vi "5. Identification.vi"() -> ()   [LabVIEW 2019, in "SJCube.lvlib"]
uses:
  SJCube.lvlib
  idState.ctl
  <vilib>/Platform/TimedLoop/XDataNode/timing_clust.ctl
  <vilib>/Platform/TimedLoop/XDataNode/nitl_modes.ctl
  <vilib>/Platform/TimedLoop/XDataNode/wakeup.ctl
  <vilib>/Platform/TimedLoop/XDataNode/XDataNode.xnode
  <vilib>/Platform/TimedLoop/XDataNode/XDNodeRunTimeDep.lvlib
panel:
  in  "Logging Setting":T1
  out "motor overswing":bool
  in  "overswing (deg)":dbl=15.0 format="%#_13g"
  out "Stick deg greater then":bool
  out "error out":errorcluster
  in  "Play Button":bool
  out "Waveform Chart":T2(graph)
  in  "Configuration Sine":T3={"Amp (Volts)"=0.4, "Freq (Hz)"=10.0, "Time (s)"=5.0, "SignalType"=enum."IdSine"} {"Amp (Volts)" scale=0.0..12.0}
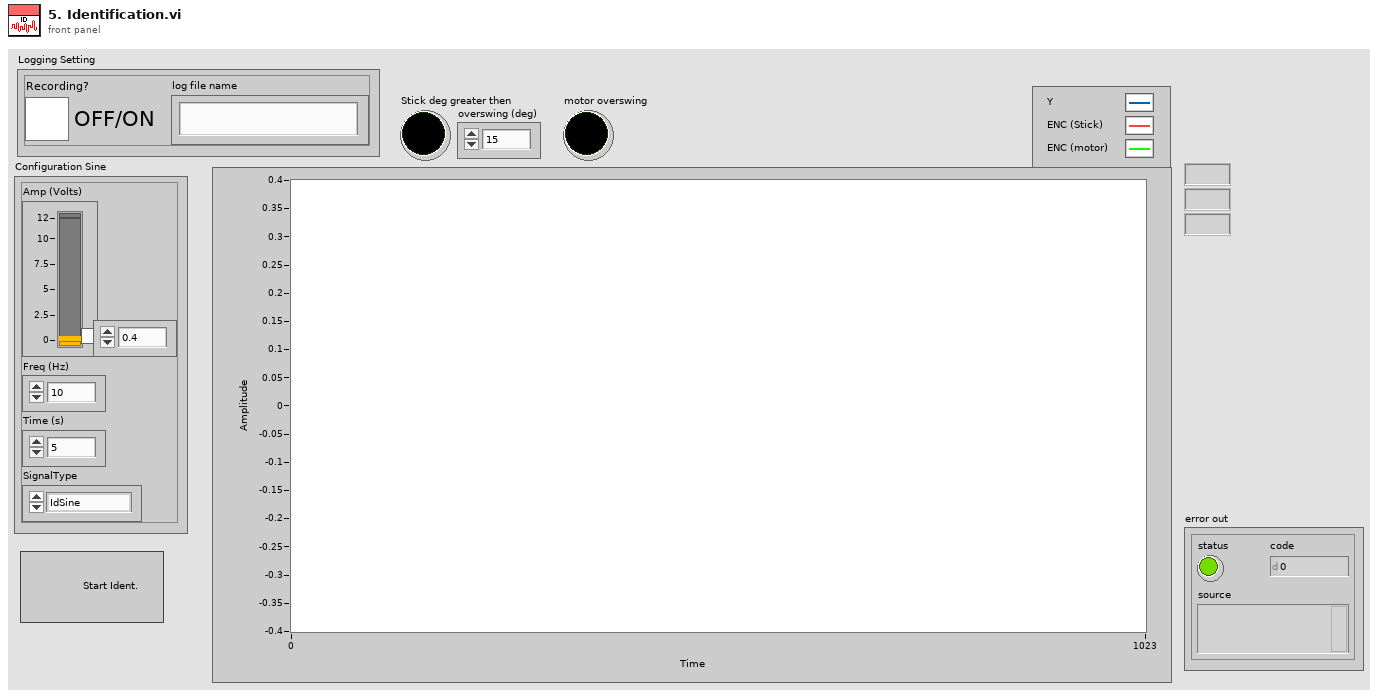
[diagram p1: front panel]
types:
  T1 = cluster{"Recording?":bool, "log file name":string}
  T2 = cluster{dbl, "StickEncoder (deg)":dbl, "MotorEncoder (deg)":dbl}
  T3 = cluster{"Amp (Volts)":dbl, "Freq (Hz)":dbl, "Time (s)":dbl, "SignalType":enum16{"IdSine", "IdSquare"}}
  T4 = typedef "SJCube.lvlib/idState.ctl" = enum16{"Configuration", "Id", "Logging", "End"}
  T5 = cluster{dbl, "StickEncoder (deg)":dbl, "MotorEncoder (deg)":dbl}[]
  T6 = typedef "XDNodeRunTimeDep.lvlib/timing_clust.ctl" = cluster{"Expected End [f-1]":u64, "Actual End [f-1]":u64, "Finished Late? [f-1]":bool, "Expected End [i-1]":u64, "Actual End [i-1]":u64, "Finished Late? [i-1]":bool, "Expected Start [i]":u64, "Actual Start [i]":u64, "Expected Start [f]":u64, "Actual Start [f]":u64, "Source Name":string, "Structure Name":string, "Period":i64, "Deadline":i64, "Offset":i64, "Start":i64, "Priority":i32, "Timeout":i32, "Mode":T7, "Wakeup Reason":T8, "Error":errorcluster, "Source Type":string, "Secondary Source Type":string, "Global End Time":u64, "Global Start Time":u64, "Frame Duration":u64, "Iteration Duration":u64, "Assigned CPU":i32, "I/O Scan Engine Mode":u32}
  T7 = typedef "XDNodeRunTimeDep.lvlib/nitl_modes.ctl" = enum32{"No Change", "Process missed periods, maintain original phase", "Discard missed periods, maintain original phase", "Process missed periods, ignore original phase", "Discard missed periods, ignore original phase"}
  T8 = typedef "XDNodeRunTimeDep.lvlib/wakeup.ctl" = enum32{"Normal", "Aborted", "Asynchronous wakeup", "Timing source error", "Timed loop error", "Timeout"}
  T9 = enum16{"open", "replace", "create", "open or create", "replace or create", "replace or create with confirmation"}
  T10 = cluster{"Amp (Volts)":dbl, "StickEncoder (deg)":dbl, "MotorEncoder (deg)":dbl}
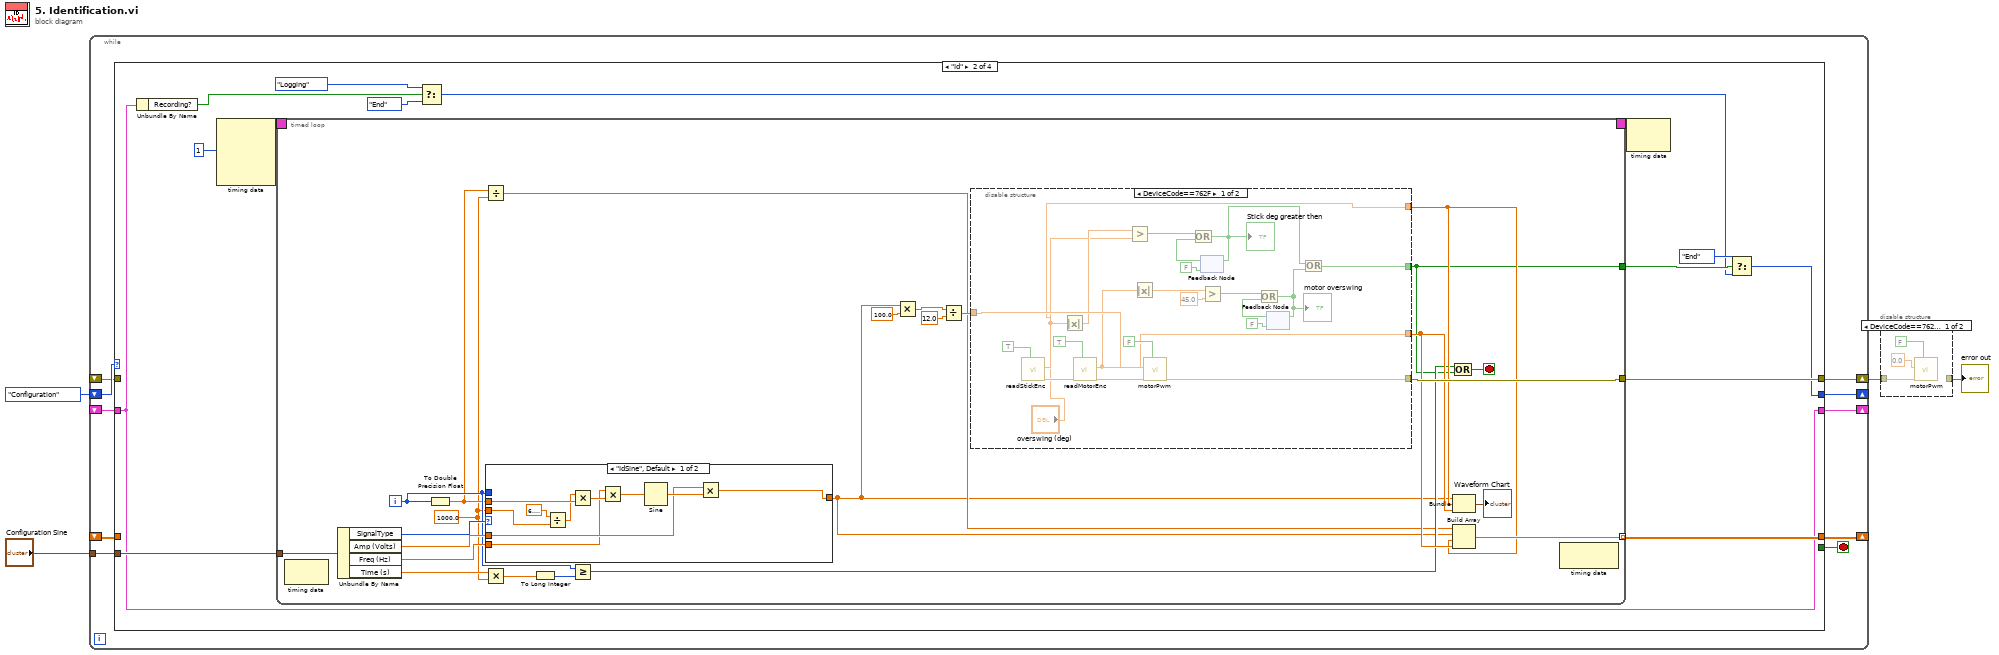
[diagram p0: block diagram]
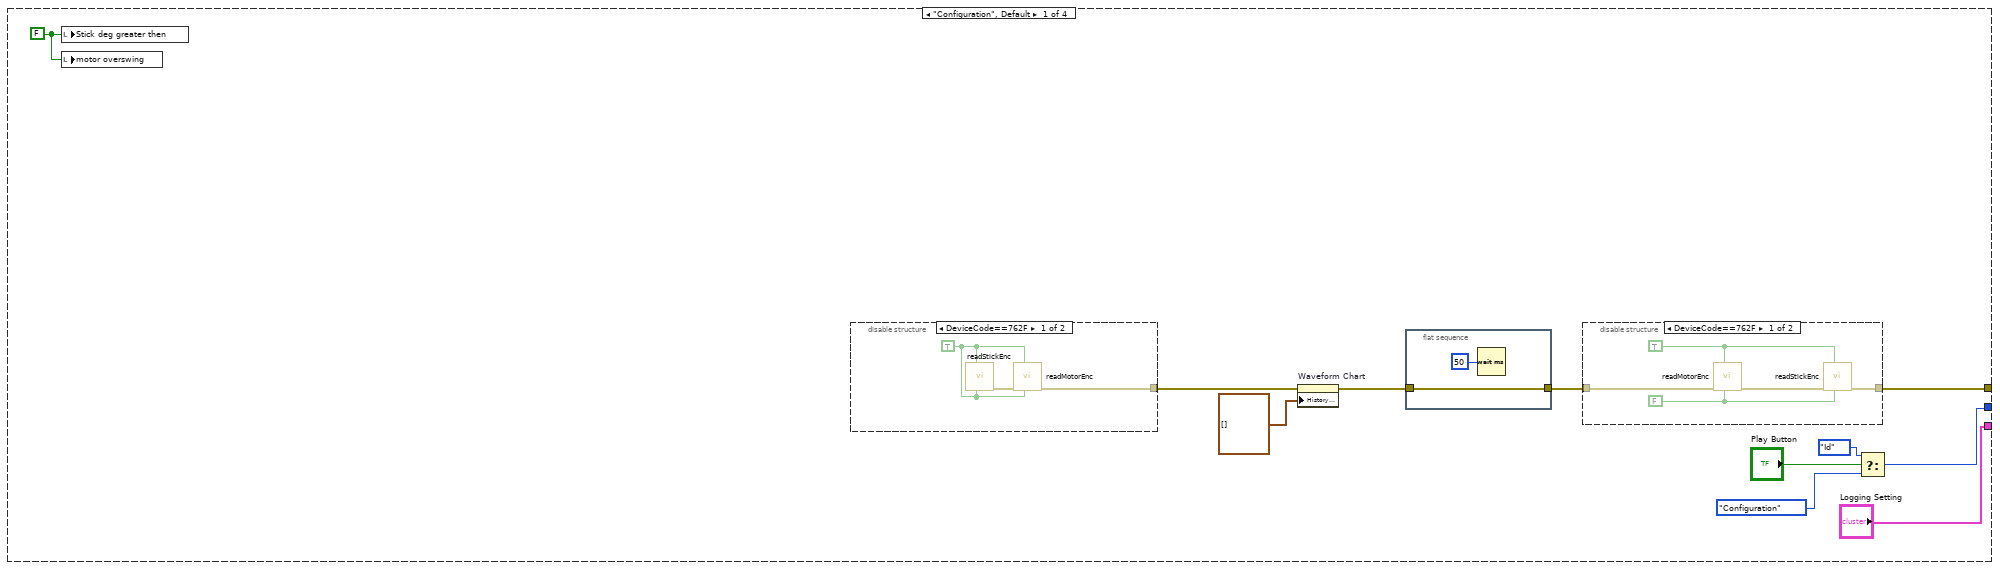
[diagram p3: hidden frame]
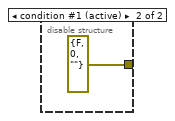
[diagram p4: hidden frame]
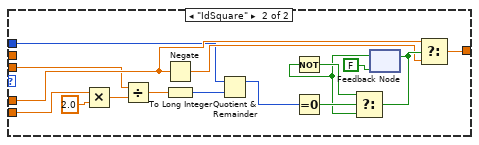
[diagram p6: hidden frame]
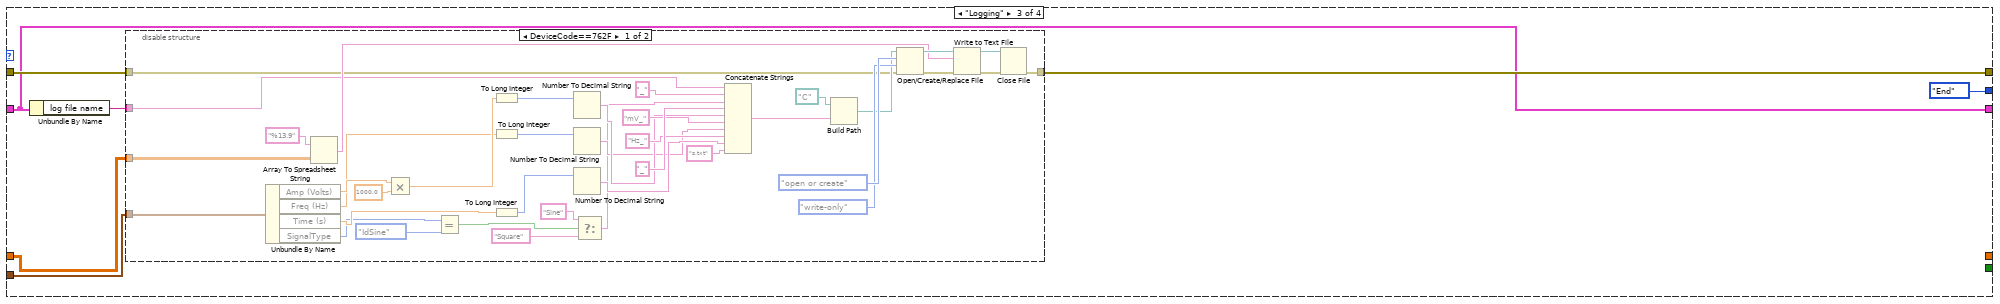
[diagram p8: hidden frame]
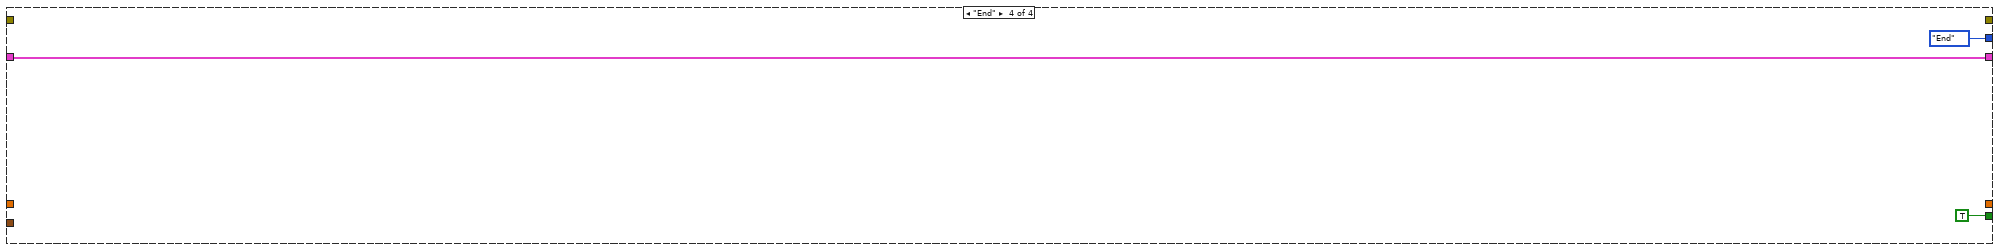
[diagram p10: hidden frame]
diagram:
  n1 = while {
    shift-right: [w12] -> _
    shift-left: _ -> [w11]
    tunnel: "Configuration Sine" -> [w10]
    shift-right: [w8] -> _
    shift-left: idState."Configuration" ("Exp. State") -> [w9]
    shift-right: [w13] -> w4
    shift-left: _ -> [w7]
    shift-right: [w6] -> _
    shift-left: _ -> [w5]
    stop <- w14 stop-if-true
    n2 = case shown="\"Id\"" w9 {
      tunnel: [_ _ _ TRUE] -> w14
      tunnel: [w21 w48 w133 _] -> w13
      tunnel: [_ w47 _ _] -> w12
      tunnel: w11 -> [_ _ w136 _]
      tunnel: w10 -> [_ w46 w132 _]
      tunnel: [w22 w44 idState."End" ("IdentificationState") idState."End" ("IdentificationState")] -> w8
      tunnel: w7 -> [_ _ w134 _]
      tunnel: ["Logging Setting" w42 w131 w175] -> w6
      tunnel: w5 -> [_ w42 w131 w175]
      frame "Configuration", Default {
        w18 = FALSE ("Stick deg greater then 15")
        n3 = local write "Stick deg greater then"(w18) -> ()
        n4 = local write "motor overswing"(w18) -> ()
        n5 = disable-structure shown="DeviceCode==762F" {
          disable-tunnel: [w28 errorcluster {"status"=FALSE, "code"=0, "source"=""} ("error out")] -> w19
          frame condition #0 {
            w29 = TRUE ("Reverse ENC?")
            n6 = call "readStickEnc.vi"("Reset Counter"=w29, "Reverse ENC?"=w29) -> ("error out"=w30:errorcluster)  [unwired: 8 in, 1 out]
            n7 = call "readMotorEnc.vi"("Reset Counter"=w29, "Reverse ENC?"=w29, "error in (no error)"=w30) -> ("error out"=w28:errorcluster)  [unwired: 7 in, 1 out]
          }
          frame condition #1 (active) {
          }
        }
        n8 = property on="Waveform Chart" class="WFChart (strict)"(error in=w19, "History Data"=T5 []) -> (error out=w16:errorcluster)  [unwired: 1 in, 1 out]
        n9 = flat-sequence {
          tunnel: [w26] -> w17
          tunnel: w16 -> [w26]
          frame #0 {
            n10 = Wait (ms)(milliseconds to wait=u32 50) -> ()  [unwired: 1 out]
          }
        }
        n11 = disable-structure shown="DeviceCode==762F" {
          disable-tunnel: [w34 w37] -> w21
          disable-tunnel: w17 -> [w33 w37]
          frame condition #0 {
            w32 = TRUE ("Reverse ENC?")
            w35 = FALSE ("Reset Counter")
            n12 = call "readMotorEnc.vi"("Reset Counter"=w35, "Reverse ENC?"=w32, "error in (no error)"=w33) -> ("error out"=w36:errorcluster)  [unwired: 7 in, 1 out]
            n13 = call "readStickEnc.vi"("Reset Counter"=w35, "Reverse ENC?"=w32, "error in (no error)"=w36) -> ("error out"=w34:errorcluster)  [unwired: 7 in, 1 out]
          }
          frame condition #1 (active) {
          }
        }
        n14 = Select(t=idState."Id" ("IdentificationState"), s="Play Button", f=idState."Configuration" ("IdentificationState")) -> (s? t:f=w22:T4)
      }
      frame "Id" {
        n15 = Unbundle By Name(w42) -> ("Recording?"=w41:bool)
        n16 = node-c288(i64 1 ("Period")) -> (w51:T6)  [unwired: 3 in]
        n17 = timed-loop {
          timing: w51 -> [_]
          timing-out: [_] -> w50
          tunnel: [w72] -> w48
          tunnel: [w69] -> w47 mode=indexing
          tunnel: w46 -> [w61]
          tunnel: [w52] -> w43
          i -> [w59]
          stop <- w56 stop-if-true
          w57 = 1000.0 ("y")
          n18 = node-c288() -> ()  [unwired: 1 in, 1 out]
          n19 = Unbundle By Name(w61) -> ("SignalType"=w60:enum16{"IdSine", "IdSquare"}, "Amp (Volts)"=w64:dbl, "Freq (Hz)"=w63:dbl, "Time (s)"=w66:dbl)
          n20 = To Double Precision Float(number=w59) -> (double precision float=w58:dbl)
          n21 = Divide(x=w58, y=w57) -> (x/y=w54:dbl)
          n22 = Multiply(x=w66, y=w57) -> (x*y=w65:dbl)
          n23 = case shown="\"IdSine\", Default" w60 {
            tunnel: w64 -> [w82 w90]
            tunnel: w63 -> [w81 w101]
            tunnel: [w80 w89] -> w53
            tunnel: w59 -> [_ w88]
            tunnel: w58 -> [w79 _]
            tunnel: w57 -> [w76 w86]
            frame "IdSine", Default {
              n24 = Divide(x=6.283185307179586, y=w76) -> (x/y=w77:dbl)
              n25 = Multiply(x=w77, y=w79) -> (x*y=w85:dbl)
              n26 = Multiply(x=w81, y=w85) -> (x*y=w84:dbl)
              n27 = Sine(x=w84) -> (sin(x)=w83:dbl)
              n28 = Multiply(x=w82, y=w83) -> (x*y=w80:dbl)
            }
            frame "IdSquare" {
              n29 = Multiply(x=w101, y=2.0) -> (x*y=w99:dbl)
              n30 = Divide(x=w86, y=w99) -> (x/y=w98:dbl)
              n31 = Negate(x=w90) -> (-x=w91:dbl)
              n32 = To Long Integer(number=w98) -> (32bit integer=w97:i32)
              n33 = Quotient & Remainder(x=w88, y=w97) -> (x-y*floor(x/y)=w96:i32)  [unwired: 1 out]
              n34 = Equal To 0?(x=w96) -> (x = 0?=w95:bool)
              n35 = feedback #1(FALSE) -> (w93:bool)
              n36 = Not(x=w93) -> (.not. x?=w94:bool)
              n37 = Select(t=w94, s=w95, f=w93) -> (s? t:f=w92:bool)
              n38 = feedback-in #1(w92) -> ()
              n39 = Select(t=w90, s=w92, f=w91) -> (s? t:f=w89:dbl)
            }
          }
          n40 = To Long Integer(number=w65) -> (32bit integer=w62:i32)
          n41 = Greater Or Equal?(x=w59, y=w62) -> (x >= y?=w55:bool)
          n42 = Multiply(x=w53, y=100.0) -> (x*y=w70:dbl)
          n43 = Divide(x=w70, y=12.0) -> (x/y=w74:dbl)
          n44 = disable-structure shown="DeviceCode==762F" {
            disable-tunnel: w74 -> [w122 _]
            disable-tunnel: [w119 _] -> w72
            disable-tunnel: [w105 _] -> w68
            disable-tunnel: [w116 _] -> w67
            disable-tunnel: [w102 _] -> w52
            frame condition #0 {
              n45 = call "readStickEnc.vi"("Reverse ENC?"=TRUE) -> ("error out"=w117:errorcluster, "StickEncoder (deg)"=w116:dbl)  [unwired: 9 in]
              n46 = Absolute Value(x=w116) -> (abs(x)=w115:dbl)
              n47 = call "readMotorEnc.vi"("Reverse ENC?"=TRUE, "error in (no error)"=w117) -> ("error out"=w120:errorcluster, "MotorEncoder (deg)"=w105:dbl)  [unwired: 8 in]
              n48 = Greater?(x=w115, y="overswing (deg)") -> (0:w113:bool)
              n49 = Absolute Value(x=w105) -> (abs(x)=w109:dbl)
              n50 = call "motorPwm.vi"("reverse?"=FALSE, "error in (no error)"=w120, "Speed (PWM)"=w122) -> ("error out"=w119:errorcluster)  [unwired: 8 in]
              n51 = feedback #2(FALSE) -> (w112:bool)
              n52 = Or(x=w113, y=w112) -> (x .or. y?=w104:bool)
              "Stick deg greater then" <- w104
              n53 = feedback-in #2(w104) -> ()
              n54 = Greater?(x=w109, y=45.0) -> (0:w107:bool)
              n55 = feedback #3(FALSE) -> (w106:bool)
              n56 = Or(x=w107, y=w106) -> (x .or. y?=w103:bool)
              "motor overswing" <- w103
              n57 = feedback-in #3(w103) -> ()
              n58 = Or(x=w104, y=w103) -> (x .or. y?=w102:bool)
            }
            frame condition #1 (active) {
            }
          }
          n59 = Bundle("Amp (Volts)"=w53, "StickEncoder (deg)"=w67, "MotorEncoder (deg)"=w68) -> (→"Waveform Chart":T10)  [unwired: 1 in]
          n60 = Build Array(w54, w53, w67, w68) -> (w69:dbl[])
          n61 = Compound Arithmetic op=OR(w55, w52) -> (w56:bool)
          n62 = node-c288() -> ()  [unwired: 1 in, 1 out]
        }
        n63 = Select(t=idState."Logging" ("IdentificationState"), s=w41, f=idState."End") -> (s? t:f=w38:T4)
        n64 = node-c288(w50) -> ()  [unwired: 1 out]
        n65 = Select(t=idState."End", s=w43, f=w38) -> (s? t:f=w44:T4)
      }
      frame "Logging" {
        n66 = Unbundle By Name(w131) -> ("log file name"=w130:string)
        n67 = disable-structure shown="DeviceCode==762F" {
          disable-tunnel: w136 -> [w168 _]
          disable-tunnel: [w162 _] -> w133
          disable-tunnel: w134 -> [w161 _]
          disable-tunnel: w132 -> [w160 _]
          disable-tunnel: w130 -> [w137 _]
          frame condition #0 {
            n68 = Unbundle By Name(w160) -> ("Amp (Volts)"=w152:dbl, "Freq (Hz)"=w148:dbl, "Time (s)"=w146:dbl, "SignalType"=w144:enum16{"IdSine", "IdSquare"})
            n69 = Array To Spreadsheet String(array=w168, 3:"%13.9" ("format string")) -> (spreadsheet string=w170:string)  [unwired: 1 in]
            n70 = Multiply(x=w152, y=1000.0) -> (x*y=w150:dbl)
            n71 = Equal?(x=w144, y=enum16{"IdSine", "IdSquare"}."IdSine") -> (x = y?=w142:bool)
            n72 = To Long Integer(number=w150) -> (32bit integer=w149:i32)
            n73 = To Long Integer(number=w148) -> (32bit integer=w147:i32)
            n74 = To Long Integer(number=w146) -> (32bit integer=w145:i32)
            n75 = Number To Decimal String(number=w149) -> (decimal integer string=w154:string)  [unwired: 1 in]
            n76 = Number To Decimal String(number=w147) -> (decimal integer string=w153:string)  [unwired: 1 in]
            n77 = Number To Decimal String(number=w145) -> (decimal integer string=w156:string)  [unwired: 1 in]
            n78 = Select(t="Sine" ("string"), s=w142, f="Square") -> (s? t:f=w138:string)
            n79 = Concatenate Strings(w137, "_" ("string"), w138, "_" ("string"), w154, "mV_" ("string"), w153, "Hz_" ("string"), w156, "s.txt" ("string")) -> (w166:string)
            n80 = Build Path(base path=path "C:/", name or relative path=w166) -> (appended path=w165:path)
            n81 = Open/Create/Replace File(file path (use dialog)=w165, error in=w161, operation (0:open)=T9."open or create", access (0:read/write)=enum16{"read/write", "read-only", "write-only"}."write-only") -> (refnum out=w171:refnum<file>, error out=w164:errorcluster)  [unwired: 2 in, 1 out]
            n82 = Write to Text File(file (use dialog)=w171, text=w170, error in=w164) -> (refnum out=w169:refnum<file>, error out=w163:errorcluster)  [unwired: 1 in, 1 out]
            n83 = Close File(refnum=w169, error in=w163) -> (error out=w162:errorcluster)  [unwired: 1 out]
          }
          frame condition #1 (active) {
          }
        }
      }
      frame "End" {
      }
    }
  }
  n84 = disable-structure shown="DeviceCode==762F" {
    disable-tunnel: w4 -> [w180 w181]
    disable-tunnel: [_ w181] -> w1
    frame condition #0 {
      n85 = call "motorPwm.vi"("reverse?"=FALSE, "error in (no error)"=w180, "Speed (PWM)"=0.0) -> ()  [unwired: 8 in, 1 out]
    }
    frame condition #1 (active) {
    }
  }
  "error out" <- w1
